vi "LoadOdorInf.vi"(11 "file path (dialog if empty)":path) -> (2 "Concentration":string[](array[string]), 3 "Odor":string[](array[string]))   [LabVIEW 2016]
uses:
  <vilib>/Utility/file.llb/Read Delimited Spreadsheet (string).vi
panel:
  out "all rows":string[][](array[string])
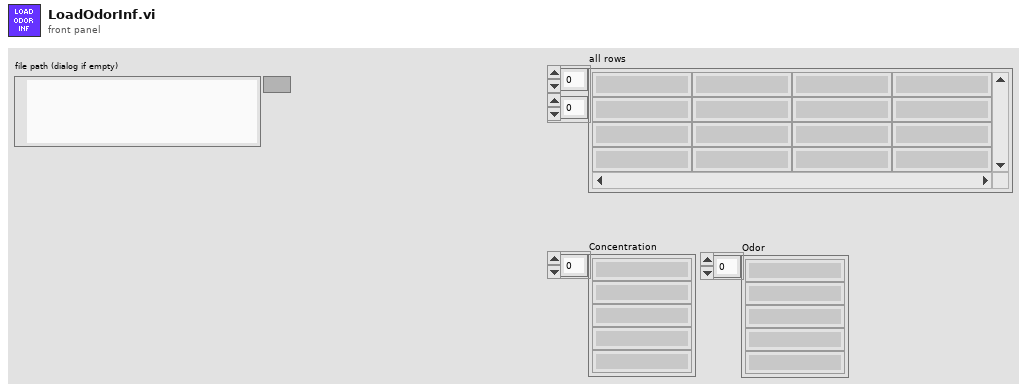
[diagram p1: front panel]
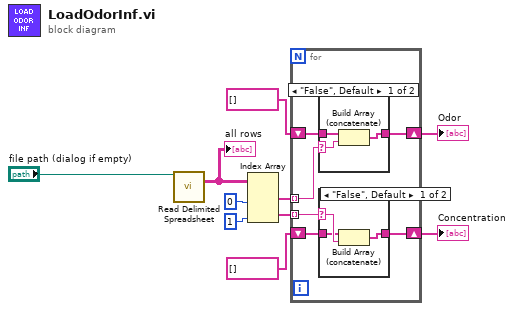
[diagram p0: block diagram]
diagram:
  n1 = call-poly <vilib>:"Read Delimited Spreadsheet.vi"("file path (dialog if empty)"="file path (dialog if empty)") -> ("all rows"=w9:string[][])  [unwired: 9 in, 5 out]
  "all rows" <- w9
  n2 = Index Array(array=w9, index (col) #1=0 ("disabled index (col)"), index (col) #2=1 ("index (col)")) -> (element #1=w6:string[], element #2=w5:string[])  [unwired: 2 in]
  n3 = for {
    tunnel: w6 -> [w16] mode=indexing
    shift-right: [w15] -> w1
    shift-left: string[] [] -> [w14]
    tunnel: w5 -> [w13] mode=indexing
    shift-right: [w12] -> w2
    shift-left: string[] [] -> [w11]
    n4 = case shown="\"False\", Default" w16 {
      selector: w16 -> [w23 _]
      tunnel: [w22 w24] -> w15
      tunnel: w14 -> [w21 w24]
      frame "False", Default {
        n5 = Build Array (concatenate)(w21, w23) -> (w22:string[])
      }
      frame "" {
      }
    }
    n6 = case shown="\"False\", Default" w13 {
      selector: w13 -> [w19 _]
      tunnel: [w18 w20] -> w12
      tunnel: w11 -> [w17 w20]
      frame "False", Default {
        n7 = Build Array (concatenate)(w17, w19) -> (w18:string[])
      }
      frame "" {
      }
    }
  }
  "Odor" <- w1
  "Concentration" <- w2
